vi "test MSS.vi"() -> ()   [LabVIEW 2023]
uses:
  Measure and Stimulus Subsystems/Measure and Stimulus Subsystems.lvclass
  Virtual Instrs/Virt Red-y Read Write/Virt Red-y Read Write.lvclass
  Configurations/Read Write CFG/Red-y Read Write CFG.lvclass
  Configurations/Red-y Read Write CFG Simulated/Red-y Read Write CFG Simulated.lvclass
panel:
  out "Output":variant
  out "Temperature":variant
  out "Flow":variant
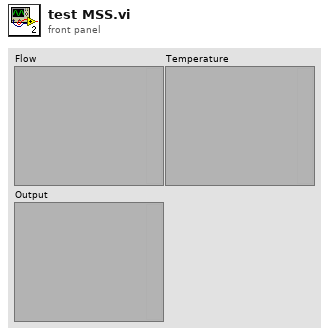
[diagram p1: front panel]
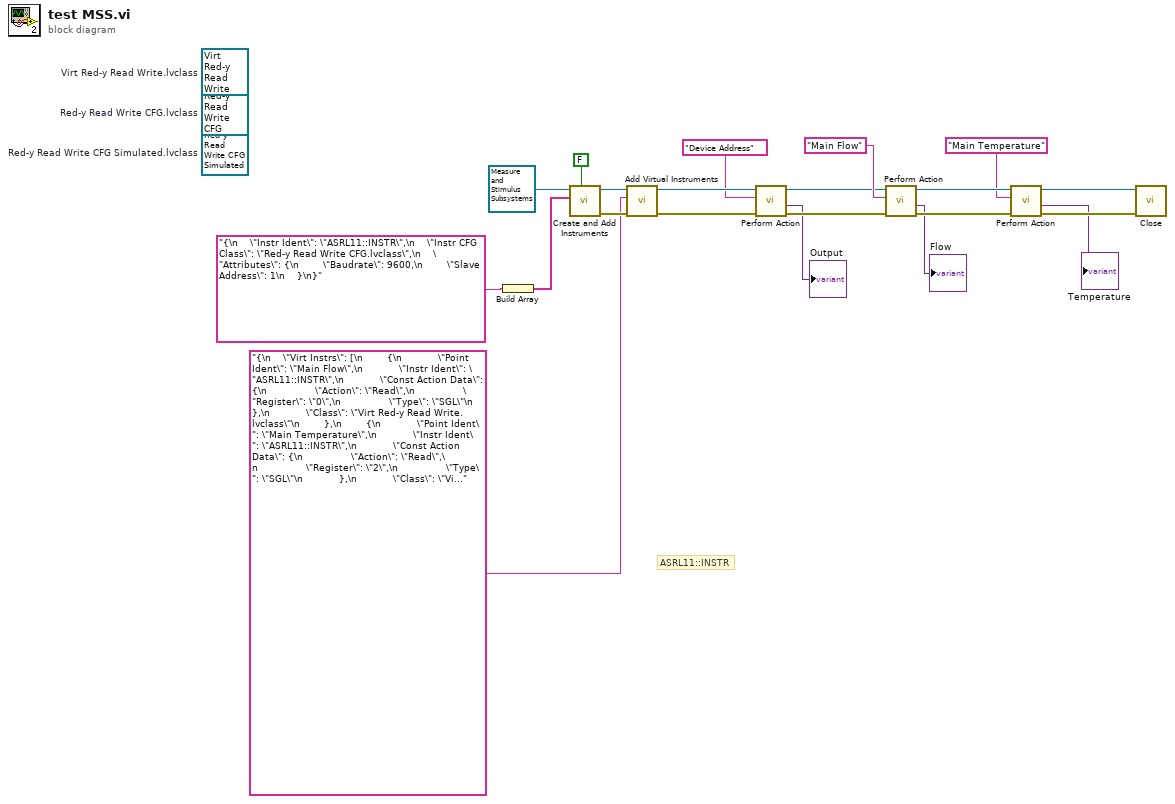
[diagram p0: block diagram]
diagram:
  (unwired) refnum<class "Red-y Read Write CFG Simulated.lvclass"> refnum  # Red-y Read Write CFG Simulated.lvclass
  (unwired) refnum<class "Red-y Read Write CFG.lvclass"> refnum  # Red-y Read Write CFG.lvclass
  (unwired) refnum<class "Virt Red-y Read Write.lvclass"> refnum  # Virt Red-y Read Write.lvclass
  # "ASRL11::INSTR"
  n1 = Build Array("{\n    \"Instr Ident\": \"ASRL11::INSTR\",\n    \"Instr CFG Class\": \"Red-y Read Write CFG.lvclass\",\n    \"Attributes\": {\n        \"Baudrate\": 9600,\n        \"Slave Address\": 1\n    }\n}") -> (w16:string[])
  n2 = call "Create and Add Instruments.vi"("Is Target?"=FALSE, "Physical Intr CFGs"=w16, "MSS in"=refnum<class "Measure and Stimulus Subsystems.lvclass"> refnum ("HAL GOOP4.lvlib:Measure and Stimulus Subsystems.lvclass")) -> ("Error Out"=w20:errorcluster, "MSS out"=w19:refnum<class "Measure and Stimulus Subsystems.lvclass">)  [unwired: 6 in, 1 out]
  n3 = call "Add Virtual Instruments.vi"("error in"=w20, "<JSON CFG>"="{\n    \"Virt Instrs\": [\n        {\n            \"Point Ident\": \"Main Flow\",\n            \"Instr Ident\": \"ASRL11::INSTR\",\n            \"Const Action Data\": {\n                \"Action\": \"Read\",\n                \"Register\": \"0\",\n                \"Type\": \"SGL\"\n            },\n            \"Class\": \"Virt Red-y Read Write.lvclass\"\n        },\n        {\n            \"Point Ident\": \"Main Temperature\",\n            \"Instr Ident\": \"ASRL11::INSTR\",\n            \"Const Action Data\": {\n                \"Action\": \"Read\",\n                \"Register\": \"2\",\n                \"Type\": \"SGL\"\n            },\n            \"Class\": \"Virt Red-y Read Write.lvclass\"\n        },\n        {\n            \"Point Ident\": \"Device Address\",\n            \"Instr Ident\": \"ASRL11::INSTR\",\n            \"Const Action Data\": {\n                \"Action\": \"Read\",\n                \"Register\": \"13\",\n                \"Type\": \"U16\"\n            },\n            \"Class\": \"Virt Red-y Read Write.lvclass\"\n        }\n    ]\n}", "MSS in"=w19) -> ("error out"=w14:errorcluster, "MSS out"=w4:refnum<class "Measure and Stimulus Subsystems.lvclass">)  [unwired: 6 in, 1 out]
  n4 = call "Perform Action.vi"("error in"=w14, "Point Ident"="Device Address", "MSS in"=w4) -> ("error out"=w5:errorcluster, "Output"=→"Output":variant, "MSS out"=w3:refnum<class "Measure and Stimulus Subsystems.lvclass">)  [unwired: 5 in, 1 out]
  n5 = call "Perform Action.vi"("error in"=w5, "Point Ident"="Main Flow" ("Task-Point Idents"), "MSS in"=w3) -> ("error out"=w13:errorcluster, "Output"=→"Flow":variant, "MSS out"=w9:refnum<class "Measure and Stimulus Subsystems.lvclass">)  [unwired: 5 in, 1 out]
  n6 = call "Perform Action.vi"("error in"=w13, "Point Ident"="Main Temperature", "MSS in"=w9) -> ("error out"=w10:errorcluster, "Output"=→"Temperature":variant, "MSS out"=w8:refnum<class "Measure and Stimulus Subsystems.lvclass">)  [unwired: 5 in, 1 out]
  n7 = call "Close.vi"("error in"=w10, "MSS in"=w8) -> ()  [unwired: 8 in, 2 out]
